vi "AIT 664 - Read Rx Ports XML.vi"(0 "Refnum in":refnum<k20>, 11 "error in (no error)":errorcluster) -> (4 "Rx Message Port":T1, 15 "error out":errorcluster)   [LabVIEW 2013, in "AIT 664 Custom Device.lvlib"]
doc: "Read RxMessagePort xml"
uses:
  AIT 664 Custom Device.lvlib
  Controls/664 - XML Rx Message Port.ctl
  Controls/664 - Sampling Type.ctl
  Controls/664 -Param.ctl
  <vilib>/xml/Close Reference(NNMap).vi
  <vilib>/xml/Close Reference(Node).vi
  <resource>/objmgr/DOMUserDefRef.rc
  <vilib>/xml/NI_XML.lvlib
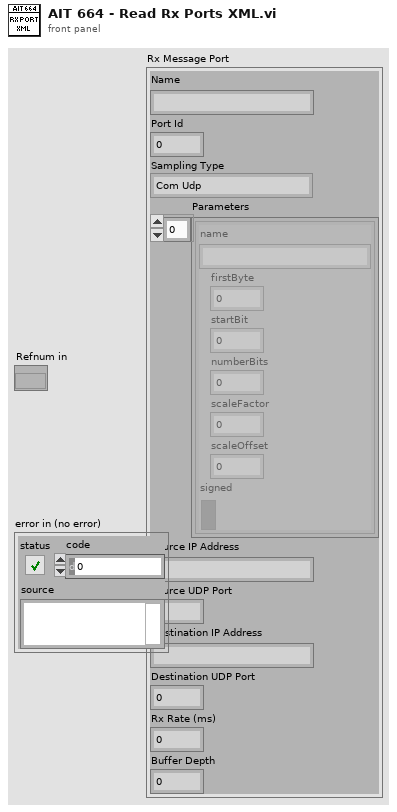
[diagram p1: front panel]
types:
  T1 = typedef "AIT 664 Custom Device.lvlib/664 - XML Rx Message Port.ctl" = cluster{"Name":string, "Port Id":u32, "Sampling Type":T2, "Parameters":T3[], "Source IP Address":string, "Source UDP Port":u32, "Destination IP Address":string, "Destination UDP Port":u32, "Rx Rate (ms)":u32, "Buffer Depth":u32}
  T2 = typedef "AIT 664 Custom Device.lvlib/664 - Sampling Type.ctl" = enum16{"Com Udp", "Com Udp Queuing", "Sap Udp", "Sap Ip", "Sap Mac", "Unknown"}
  T3 = typedef "AIT 664 Custom Device.lvlib/664 -Param.ctl" = cluster{"name":string, "firstByte":i32, "startBit":i32, "numberBits":i32, "scaleFactor":dbl, "scaleOffset":dbl, "signed":bool}
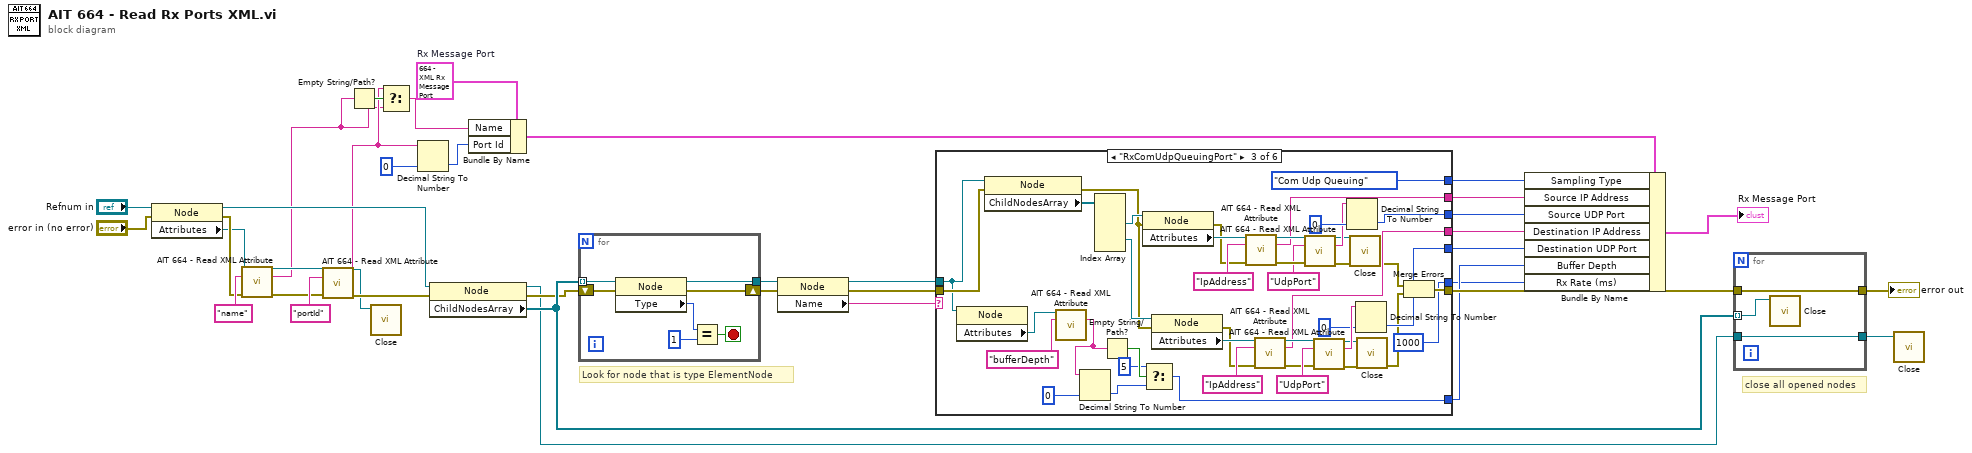
[diagram p0: block diagram]
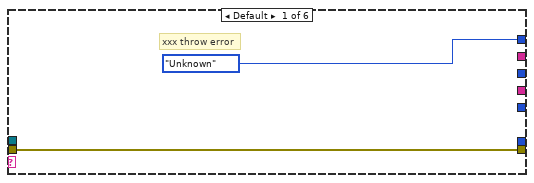
[diagram p2: hidden frame]
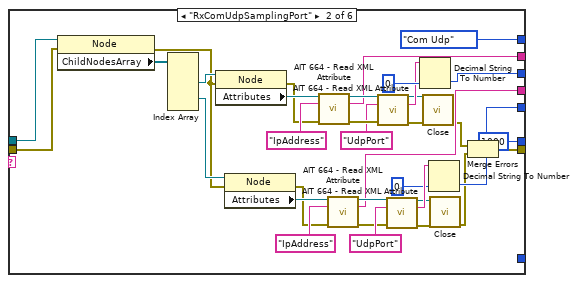
[diagram p3: hidden frame]
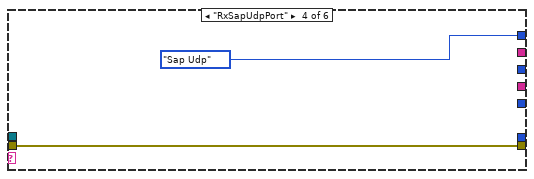
[diagram p4: hidden frame]
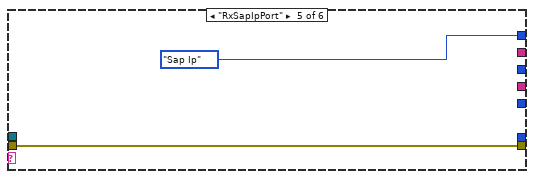
[diagram p5: hidden frame]
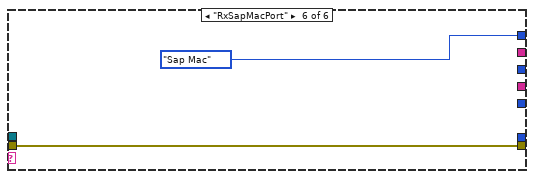
[diagram p6: hidden frame]
diagram:
  w28 = T1 {"Name"="", "Port Id"=0, "Sampling Type"=enum."Com Udp", "Parameters"=[], "Source IP Address"="", "Source UDP Port"=0, "Destination IP Address"="", "Destination UDP Port"=0, "Rx Rate (ms)"=0, "Buffer Depth"=0}  # Rx Message Port
  # "close all opened nodes"
  # "Look for node that is type ElementNode"
  n1 = property class="Node"(reference="Refnum in", error in="error in (no error)") -> (reference out=w29:refnum<k20>, error out=w22:errorcluster, "Attributes"=w21:refnum<k20>)
  n2 = call "AIT 664 - Read XML Attribute.vi"("Attributes In"=w21, "Attribute Name"="name", "error in (no error)"=w22) -> ("Attributes Out"=w25:refnum<k20>, "Attribute Text"=w4:string, "error out"=w24:errorcluster)  [unwired: 10 in]
  n3 = call "AIT 664 - Read XML Attribute.vi"("Attributes In"=w25, "Attribute Name"="portId", "error in (no error)"=w24) -> ("Attributes Out"=w27:refnum<k20>, "Attribute Text"=w5:string, "error out"=w30:errorcluster)  [unwired: 10 in]
  n4 = Empty String/Path?(string/path=w4) -> (empty?=w6:bool)
  n5 = call-poly <vilib>:"Close.vi"("named node map"=w27) -> ()  [unwired: 8 in, 1 out]
  n6 = Select(t=w5, s=w6, f=w4) -> (s? t:f=w3:string)
  n7 = Decimal String To Number(string=w5, default (0L)=u32 0 ("default (0 I32)")) -> (number=w7:u32)  [unwired: 1 in, 1 out]
  n8 = property class="Node"(reference=w29, error in=w30) -> (reference out=w18:refnum<k20>, error out=w35:errorcluster, "ChildNodesArray"=w38:refnum<k20>[])
  n9 = Bundle By Name(cluster=w28, "Name"=w3, "Port Id"=w7) -> (w31:T1)
  n10 = for {
    tunnel: w38 -> [w45] mode=indexing
    tunnel: [w41] -> w34
    shift-right: [w39] -> w36
    shift-left: w35 -> [w40]
    stop <- w44 stop-if-true
    n11 = property class="Node"(reference=w45, error in=w40) -> (reference out=w41:refnum<k20>, error out=w39:errorcluster, "Type"=w42:i32)
    n12 = Equal?(x=w42, y=1) -> (x = y?=w44:bool)
  }
  n13 = property class="Node"(reference=w34, error in=w36) -> (reference out=w13:refnum<k20>, error out=w15:errorcluster, "Name"=w37:string)
  n14 = case shown="\"RxComUdpQueuingPort\"" w37 {
    tunnel: [664_-_Sampling_Type."Unknown" ("Sampling Type") 664_-_Sampling_Type."Com Udp" ("Sampling Type") 664_-_Sampling_Type."Com Udp Queuing" ("Sampling Type") 664_-_Sampling_Type."Sap Udp" ("Sampling Type") 664_-_Sampling_Type."Sap Ip" ("Sampling Type") 664_-_Sampling_Type."Sap Mac" ("Sampling Type")] -> w32
    tunnel: w15 -> [w46 w50 w99 w126 w128 w130]
    tunnel: [w46 w49 w95 w126 w128 w130] -> w14
    tunnel: w13 -> [_ w81 w92 _ _ _]
    tunnel: [_ w65 w109 _ _ _] -> w12
    tunnel: [_ w64 w108 _ _ _] -> w11
    tunnel: [_ w63 w107 _ _ _] -> w10
    tunnel: [_ w62 w106 _ _ _] -> w9
    tunnel: [_ _ w84 _ _ _] -> w2
    tunnel: [_ u32 1000 ("Rx Rate (ms)") u32 1000 ("Rx Rate (ms)") _ _ _] -> w1
    frame Default {
      # "xxx throw error"
    }
    frame "RxComUdpSamplingPort" {
      n15 = property class="Node"(reference=w81, error in=w50) -> (error out=w55:errorcluster, "ChildNodesArray"=w73:refnum<k20>[])  [unwired: 1 out]
      n16 = Index Array(array=w73) -> (element #2=w57:refnum<k20>, element #4=w56:refnum<k20>)  [unwired: 5 in, 3 out]
      n17 = property class="Node"(reference=w57, error in=w55) -> (error out=w53:errorcluster, "Attributes"=w80:refnum<k20>)  [unwired: 1 out]
      n18 = property class="Node"(reference=w56, error in=w55) -> (error out=w54:errorcluster, "Attributes"=w66:refnum<k20>)  [unwired: 1 out]
      n19 = call "AIT 664 - Read XML Attribute.vi"("Attributes In"=w80, "Attribute Name"="IpAddress", "error in (no error)"=w53) -> ("Attributes Out"=w78:refnum<k20>, "Attribute Text"=w65:string, "error out"=w77:errorcluster)  [unwired: 10 in]
      n20 = call "AIT 664 - Read XML Attribute.vi"("Attributes In"=w66, "Attribute Name"="IpAddress", "error in (no error)"=w54) -> ("Attributes Out"=w68:refnum<k20>, "Attribute Text"=w63:string, "error out"=w69:errorcluster)  [unwired: 10 in]
      n21 = call "AIT 664 - Read XML Attribute.vi"("Attributes In"=w78, "Attribute Name"="UdpPort", "error in (no error)"=w77) -> ("Attributes Out"=w60:refnum<k20>, "Attribute Text"=w74:string, "error out"=w61:errorcluster)  [unwired: 10 in]
      n22 = call "AIT 664 - Read XML Attribute.vi"("Attributes In"=w68, "Attribute Name"="UdpPort", "error in (no error)"=w69) -> ("Attributes Out"=w58:refnum<k20>, "Attribute Text"=w72:string, "error out"=w59:errorcluster)  [unwired: 10 in]
      n23 = Decimal String To Number(string=w74, default (0L)=u32 0 ("default (0 I32)")) -> (number=w64:u32)  [unwired: 1 in, 1 out]
      n24 = call-poly <vilib>:"Close.vi"("error in (no error)"=w61, "named node map"=w60) -> ("error out"=w52:errorcluster)  [unwired: 7 in]
      n25 = Decimal String To Number(string=w72, default (0L)=u32 0 ("default (0 I32)")) -> (number=w62:u32)  [unwired: 1 in, 1 out]
      n26 = call-poly <vilib>:"Close.vi"("error in (no error)"=w59, "named node map"=w58) -> ("error out"=w51:errorcluster)  [unwired: 7 in]
      n27 = Merge Errors(w52, w51) -> (w49:errorcluster)
    }
    frame "RxComUdpQueuingPort" {
      n28 = property class="Node"(reference=w92) -> ("Attributes"=w91:refnum<k20>)  [unwired: 1 in, 2 out]
      n29 = property class="Node"(reference=w92, error in=w99) -> (error out=w98:errorcluster, "ChildNodesArray"=w117:refnum<k20>[])  [unwired: 1 out]
      n30 = call "AIT 664 - Read XML Attribute.vi"("Attributes In"=w91, "Attribute Name"="bufferDepth") -> ("Attribute Text"=w86:string)  [unwired: 11 in, 2 out]
      n31 = Decimal String To Number(string=w86, default (0L)=u32 0 ("default (0 I32)")) -> (number=w85:u32)  [unwired: 1 in, 1 out]
      n32 = Index Array(array=w117) -> (element #2=w101:refnum<k20>, element #4=w100:refnum<k20>)  [unwired: 5 in, 3 out]
      n33 = Empty String/Path?(string/path=w86) -> (empty?=w90:bool)
      n34 = property class="Node"(reference=w101, error in=w98) -> (error out=w97:errorcluster, "Attributes"=w124:refnum<k20>)  [unwired: 1 out]
      n35 = Select(t=u32 5 ("default (0 I32)"), s=w90, f=w85) -> (s? t:f=w84:u32)
      n36 = property class="Node"(reference=w100, error in=w98) -> (error out=w96:errorcluster, "Attributes"=w110:refnum<k20>)  [unwired: 1 out]
      n37 = call "AIT 664 - Read XML Attribute.vi"("Attributes In"=w124, "Attribute Name"="IpAddress", "error in (no error)"=w97) -> ("Attributes Out"=w122:refnum<k20>, "Attribute Text"=w109:string, "error out"=w121:errorcluster)  [unwired: 10 in]
      n38 = call "AIT 664 - Read XML Attribute.vi"("Attributes In"=w110, "Attribute Name"="IpAddress", "error in (no error)"=w96) -> ("Attributes Out"=w112:refnum<k20>, "Attribute Text"=w107:string, "error out"=w113:errorcluster)  [unwired: 10 in]
      n39 = call "AIT 664 - Read XML Attribute.vi"("Attributes In"=w122, "Attribute Name"="UdpPort", "error in (no error)"=w121) -> ("Attributes Out"=w104:refnum<k20>, "Attribute Text"=w118:string, "error out"=w105:errorcluster)  [unwired: 10 in]
      n40 = call "AIT 664 - Read XML Attribute.vi"("Attributes In"=w112, "Attribute Name"="UdpPort", "error in (no error)"=w113) -> ("Attributes Out"=w102:refnum<k20>, "Attribute Text"=w116:string, "error out"=w103:errorcluster)  [unwired: 10 in]
      n41 = Decimal String To Number(string=w118, default (0L)=u32 0 ("default (0 I32)")) -> (number=w108:u32)  [unwired: 1 in, 1 out]
      n42 = call-poly <vilib>:"Close.vi"("error in (no error)"=w105, "named node map"=w104) -> ("error out"=w94:errorcluster)  [unwired: 7 in]
      n43 = Decimal String To Number(string=w116, default (0L)=u32 0 ("default (0 I32)")) -> (number=w106:u32)  [unwired: 1 in, 1 out]
      n44 = call-poly <vilib>:"Close.vi"("error in (no error)"=w103, "named node map"=w102) -> ("error out"=w93:errorcluster)  [unwired: 7 in]
      n45 = Merge Errors(w94, w93) -> (w95:errorcluster)
    }
    frame "RxSapUdpPort" {
    }
    frame "RxSapIpPort" {
    }
    frame "RxSapMacPort" {
    }
  }
  n46 = Bundle By Name(cluster=w31, "Sampling Type"=w32, "Source IP Address"=w12, "Source UDP Port"=w11, "Destination IP Address"=w10, "Destination UDP Port"=w9, "Buffer Depth"=w2, "Rx Rate (ms)"=w1) -> (→"Rx Message Port":T1)
  n47 = for {
    tunnel: w14 -> [w133]
    tunnel: w38 -> [w134] mode=indexing
    tunnel: [w133] -> w16
    tunnel: w18 -> [w132]
    tunnel: [w132] -> w17
    n48 = call-poly <vilib>:"Close.vi"("node"=w134) -> ()  [unwired: 8 in, 1 out]
  }
  "error out" <- w16
  n49 = call-poly <vilib>:"Close.vi"("node"=w17) -> ()  [unwired: 8 in, 1 out]
